vi "DeleteRoomTable.vi"(8 "error in":errorcluster) -> (0 "error out":errorcluster)   [LabVIEW 2015, in "DatabaseApi.lvlib"]
uses:
  DatabaseApi.lvlib
  TypeDef/Room/RoomTableDbTableName.ctl
  <vilib>/addons/database/Connection.llb/DB Tools Open Connec (Path).vi
  <vilib>/addons/database/NI_Database_API.lvlib
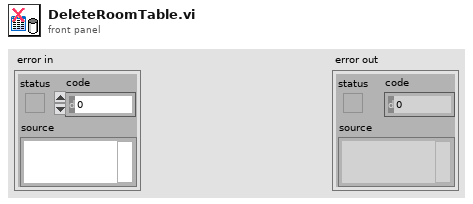
[diagram p1: front panel]
types:
  T1 = typedef "DatabaseApi.lvlib/RoomTableDbTableName.ctl" = string
  T2 = typedef "NI_Database_API.lvlib/Conn ObjectReference.ctl" = refnum<k1>
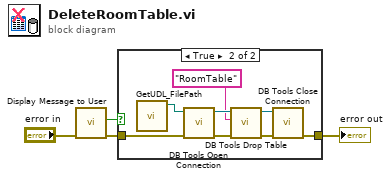
[diagram p0: block diagram]
diagram:
  n1 = call "Display Message to User"("error in (no error)"="error in") -> ("error out"=w2:errorcluster, "OK"=w1:bool)  [unwired: 9 in]
  n2 = case shown="True" w1 {
    tunnel: [w5 w7] -> w4
    tunnel: w2 -> [w5 w6]
    frame False {
    }
    frame True {
      n3 = call "GetUDL_FilePath.vi"() -> ("UDL file path"=w13:path)  [unwired: 11 in]
      n4 = call-poly <vilib>:"DB Tools Open Connection.vi"("error in (no error)"=w6, "connection information"=w13) -> ("error out"=w9:errorcluster, "connection reference"=w10:T2)  [unwired: 6 in]
      n5 = call <vilib>:"DB Tools Drop Table.vi"("error in (no error)"=w9, "table"=T1 "RoomTable", "connection reference"=w10) -> ("error out"=w11:errorcluster, "connection reference out"=w12:T2)  [unwired: 5 in]
      n6 = call <vilib>:"DB Tools Close Connection.vi"("error in (no error)"=w11, "connection reference"=w12) -> ("error out"=w7:errorcluster)  [unwired: 5 in]
    }
  }
  "error out" <- w4
